vi "RemIO Module UI.vi"(8 "error in (no error)":errorcluster, 11 "Node Ptr":T1 format="%.0x") -> (0 "error out":errorcluster)   [LabVIEW 2019, in "Modules.lvlib" / "RemIO Module.lvclass"]
uses:
  RemIO Module.lvclass
  <vilib>/NI VeriStand/Custom Device API/Custom Device Item Ref.ctl
  RSI Module/SubPanel Command.ctl
  <vilib>/NI VeriStand/Custom Device API/Custom Device API.lvlib
  RSI Module/RSI Module.lvclass
panel:
  in  "SubPanel Event":refnum<user-event>
  in  "Header":cluster{"Section Name":string}={"Section Name"="Custom Device Item Settings"}
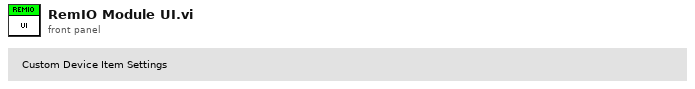
[diagram p1: front panel]
types:
  T1 = typedef "Custom Device API.lvlib/Custom Device Item Ref.ctl" = u64
  T2 = typedef "Modules.lvlib/RSI Module.lvclass/SubPanel Command.ctl" = enum16{"Stop"}
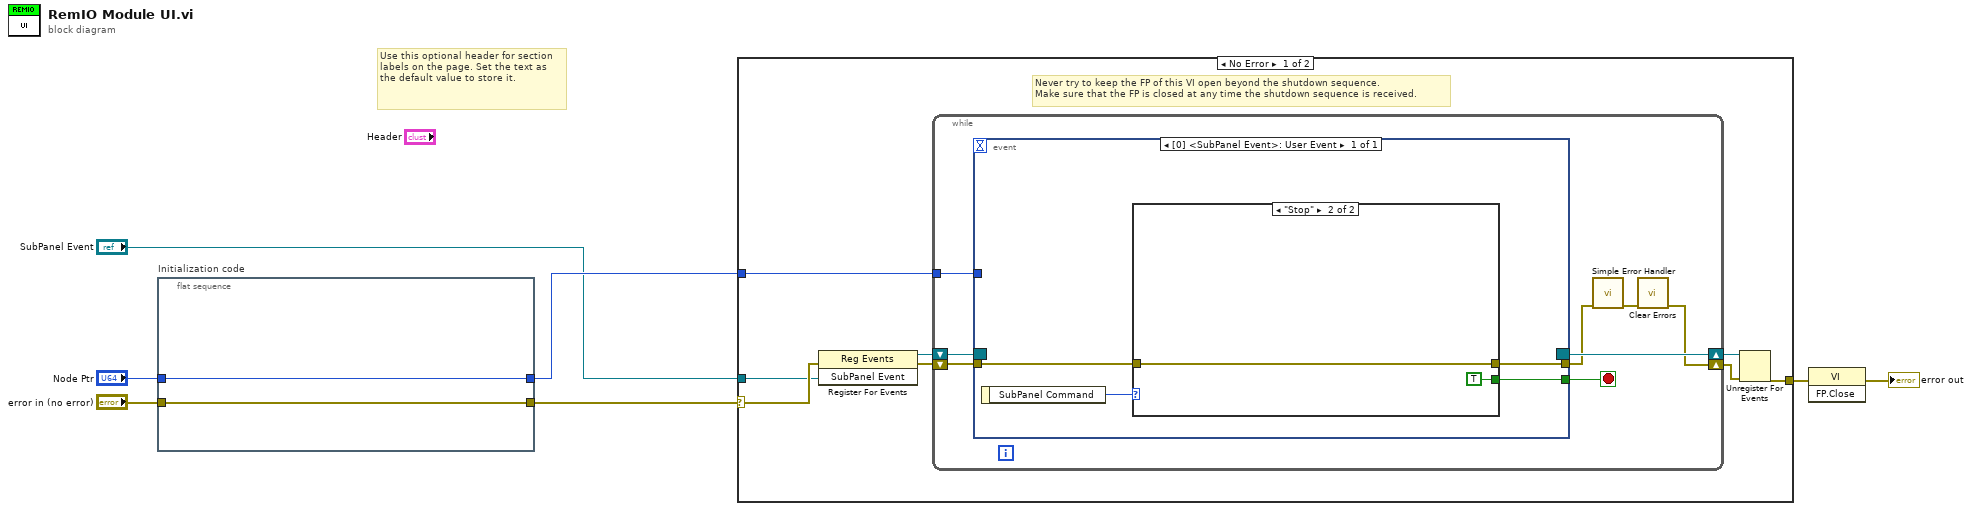
[diagram p0: block diagram]
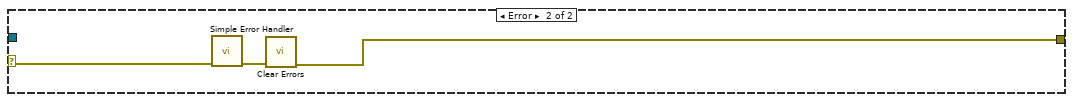
[diagram p3: hidden frame]
diagram:
  # "Use this optional header for section labels on the page. Set the text as the default value to store it."
  n1 = flat-sequence "Initialization code" {
    tunnel: "error in (no error)" -> [w8]
    tunnel: "Node Ptr" -> [w9]
    tunnel: [w8] -> w1
    tunnel: [w9] -> w4
    frame #0 {
    }
  }
  n2 = case shown="No Error" w1 {
    selector: w1 -> [w11 w35]
    tunnel: [w15 w33] -> w7
    tunnel: w4 -> [w12 _]
    tunnel: "SubPanel Event" -> [w10 _]
    frame No Error {
      # "Never try to keep the FP of this VI open beyond the shutdown sequence.\nMake sure that the FP is closed at any time the shutdown sequence is received."
      n3 = register-events(error in=w11, w10) -> (reference out=w13:refnum<event-registration>, error out=w14:errorcluster)  [unwired: 1 in]
      n4 = while {
        tunnel: w12 -> [w21]
        shift-right: [w18] -> w16
        shift-left: w14 -> [w24]
        shift-right: [w25] -> w17
        shift-left: w13 -> [w23]
        stop <- w22 stop-if-true
        n5 = event shown="[0] <SubPanel Event>: User Event" {
          selector: w23 -> [_]
          dyn-events: [_] -> w25
          timeout: _ -> [_]
          tunnel: w24 -> [w28]
          tunnel: [w26] -> w22
          tunnel: [w27] -> w20
          tunnel: w21 -> [_]
          event User Event {
            n6 = event-data() -> ("SubPanel Command"=w29:T2)  [unwired: 1 out]
            n7 = case shown="\"Stop\"" w29 {
              tunnel: w28 -> [w30 w31]
              tunnel: [w30 w31] -> w27
              tunnel: [_ TRUE] -> w26
              frame Default {
              }
              frame "Stop" {
              }
            }
          }
        }
        n8 = call <vilib>:"Simple Error Handler.vi"("error in (no error)"=w20) -> ("error out"=w19:errorcluster)  [unwired: 1 in, 7 out]
        n9 = call <vilib>:"Clear Errors.vi"("error in (no error)"=w19) -> ("error out"=w18:errorcluster)  [unwired: 1 in, 5 out]
      }
      n10 = Unregister For Events(event registration refnum=w17, error in=w16) -> (error out=w15:errorcluster)
    }
    frame Error {
      n11 = call <vilib>:"Simple Error Handler.vi"("error in (no error)"=w35) -> ("error out"=w34:errorcluster)  [unwired: 1 in, 7 out]
      n12 = call <vilib>:"Clear Errors.vi"("error in (no error)"=w34) -> ("error out"=w33:errorcluster)  [unwired: 1 in, 5 out]
    }
  }
  n13 = invoke class="VI" method="FP.Close"(error in=w7) -> (error out=→"error out":errorcluster)  [unwired: 2 in, 2 out]
